vi "teste-noise.vi"() -> ()   [LabVIEW 2014]
uses:
  <vilib>/Utility/file.llb/Read From Spreadsheet File (DBL).vi
  <vilib>/Analysis/NI_AALBase.lvlib
panel:
  in  "separator (point) - (coma)":bool
  out "error (%)":dbl=0.04847431119267763
  out "variance":dbl=1.6232919191919618e-06 format="%0.6f"
  out "standard deviation":dbl=0.001274084737838093 format="%0.6f"
  out "mean":dbl=2.628371 format="%0.6f"
  out "Waveform Graph":dbl[](graph)=[2.6269, 2.6282, 2.6283, 2.6268, 2.6289, 2.6291, 2.6286, 2.6254, 2.6296, 2.6288, 2.6311, 2.628, 2.6263, 2.6295, 2.6308, 2.6301, 2.6281, 2.6279, 2.6295, 2.6287, 2.6293, 2.6276, 2.63, 2.6275, 2.6288, 2.627, 2.6251, 2.6283, 2.6305, 2.6283, 2.6283, 2.6279, 2.6297, 2.6294, 2.6265, 2.6268, 2.6306, 2.6294, 2.6291, 2.6275, 2.6274, 2.629, 2.6278, 2.6263, 2.6282, 2.6276, 2.6285, 2.6269, 2.6264, 2.6258, 2.6274, 2.6286, 2.6279, 2.6283, 2.6291, 2.6281, 2.6275, 2.6284, 2.6291, 2.6296, 2.6291, 2.6286, 2.6268, 2.6299, 2.6298, 2.6278, 2.6272, 2.6293, 2.6282, 2.6297, 2.6294, 2.627, 2.6275, 2.6305, 2.6282, 2.628, 2.6285, 2.6302, 2.6282, 2.6276, 2.6264, 2.6282, 2.6304, 2.6295, 2.6266, 2.6268, 2.6301, 2.6287, 2.6279, 2.6293, 2.6289, 2.6292, 2.6277, 2.6288, 2.6267, 2.6305, 2.6265, 2.6294, 2.6297, 2.6282]
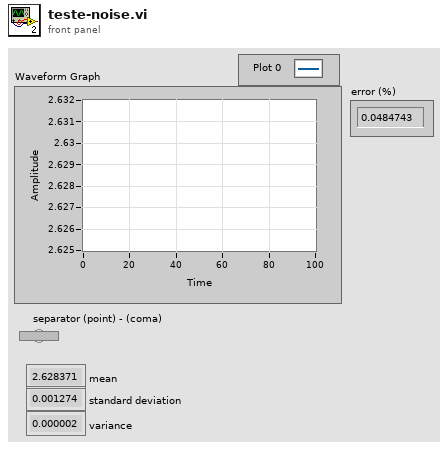
[diagram p1: front panel]
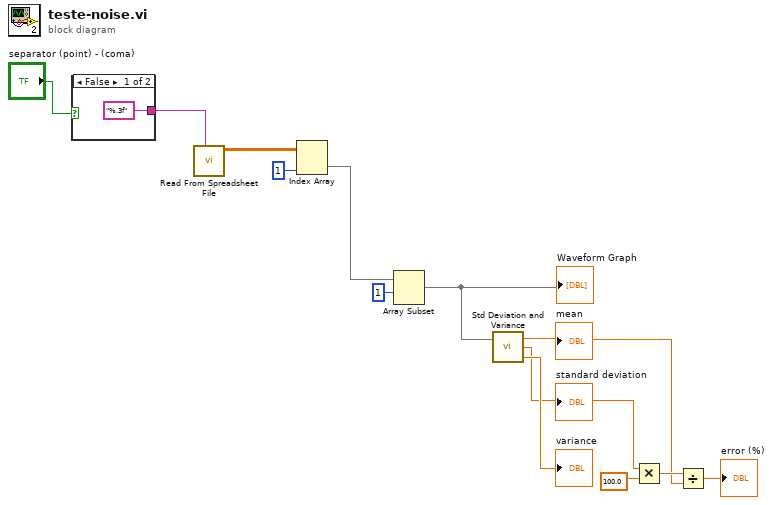
[diagram p0: block diagram]
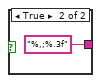
[diagram p2: hidden frame]
diagram:
  n1 = case shown="False" "separator (point) - (coma)" {
    tunnel: ["%.3f" ("format (%.3f)") "%,;%.3f" ("format (%.3f)")] -> w1
    frame False {
    }
    frame True {
    }
  }
  n2 = call-poly <vilib>:"Read From Spreadsheet File.vi"("format (%.3f)"=w1) -> ("all rows"=w13:dbl[][])  [unwired: 6 in, 4 out]
  n3 = Index Array(array=w13, index (col)=1 ("index (row)")) -> (element=w11:dbl[])  [unwired: 1 in]
  n4 = Array Subset(array=w11, index=1) -> (w9:dbl[])  [unwired: 1 in]
  "Waveform Graph" <- w9
  n5 = call <vilib>:"Std Deviation and Variance.vi"("X"=w9) -> ("mean"=w3:dbl, "standard deviation"=w4:dbl, "variance"=→"variance":dbl)  [unwired: 1 in]
  "mean" <- w3
  "standard deviation" <- w4
  n6 = Multiply(x=w4, y=100.0) -> (x*y=w6:dbl)
  n7 = Divide(x=w6, y=w3) -> (x/y=→"error (%)":dbl)
